vi "Queue_FGV.vi"(8 "error in":errorcluster, 10 "Action":T1, 11 "Queue In":refnum<queue>) -> (0 "error out":errorcluster, 3 "Queue Out":refnum<queue>)   [LabVIEW 2020]
doc: "This is the FGV VI for the Queue of this module."
uses:
  Controls/Queue.ctl
  Controls/Queue_Mode.ctl
  Controls/Queue_Action.ctl
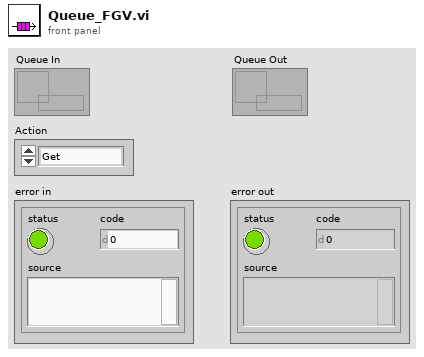
[diagram p1: front panel]
types:
  T1 = typedef "Queue_Action.ctl" = enum16{"Get", "Set", "Release"}
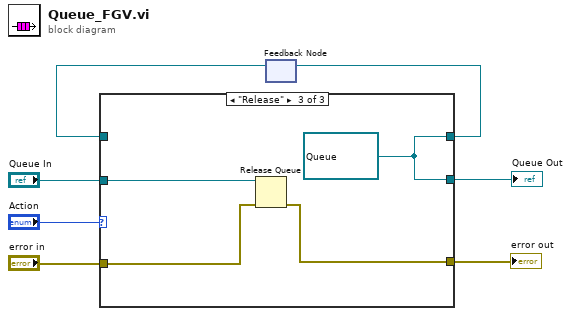
[diagram p0: block diagram]
diagram:
  n1 = feedback #1() -> (w2:refnum<queue>)  [unwired: 1 in]
  n2 = case shown="\"Release\"" "Action" {
    tunnel: "Queue In" -> [_ w11 w15]
    tunnel: [w9 w11 w12] -> w3
    tunnel: [w8 w10 w14] -> w5
    tunnel: "error in" -> [w8 w10 w13]
    tunnel: w2 -> [w9 _ _]
    tunnel: [w9 w11 w12] -> w1
    frame "Get", Default {
    }
    frame "Set" {
    }
    frame "Release" {
      w12 = refnum<queue> refnum ("queue out")
      n3 = Release Queue(queue=w15, error in (no error)=w13) -> (error out=w14:errorcluster)  [unwired: 1 in, 2 out]
    }
  }
  "error out" <- w5
  "Queue Out" <- w1
  n4 = feedback-in #1(w3) -> ()
